vi "Load Configuration.vi"(8 "error in":errorcluster, 11 "Config path":path=path "C:/GitHub/OOP_OPC UA/Config/INI Config.ini") -> (0 "error out":errorcluster)   [LabVIEW 2021]
uses:
  Controls/Channels.ctl
  Controls/Instrument.ctl
  Controls/DUT.ctl
  <vilib>/Utility/config.llb/Read Key (String).vi
  <vilib>/Utility/config.llb/NI_LVConfig.lvlib
panel:
  out "data":T1[](array[typedef])
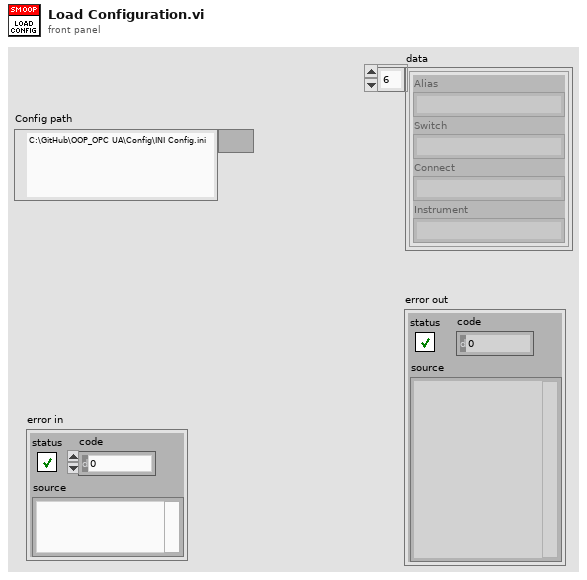
[diagram p1: front panel]
types:
  T1 = typedef "Channels.ctl" = cluster{"Alias":string, "Switch":string, "Connect":string, "Instrument":string}
  T2 = typedef "NI_LVConfig.lvlib/Config Data RefNum.ctl" = refnum<k1>
  T3 = typedef "Instrument.ctl" = cluster{"Alias":string, "VISA Resource":string, "Class":string}
  T4 = typedef "DUT.ctl" = cluster{"Alias":string, "Instrument":string, "Channel":string}
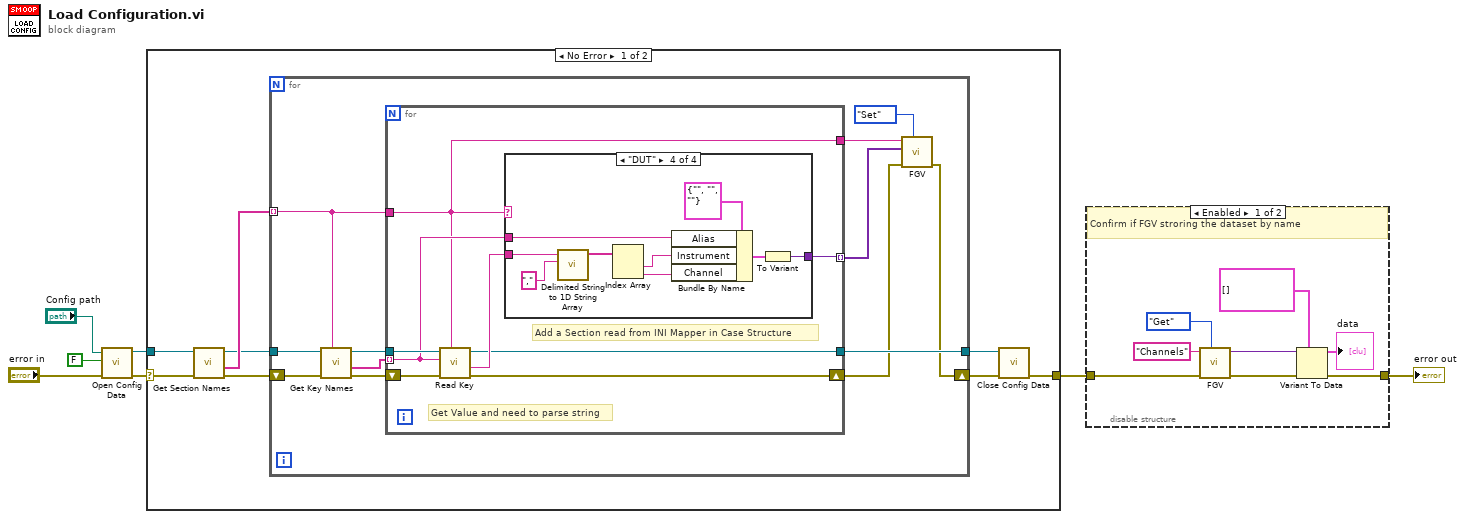
[diagram p0: block diagram]
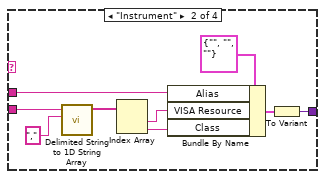
[diagram p3: hidden frame]
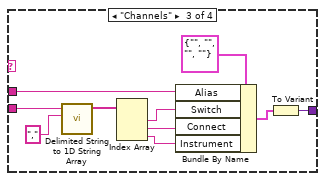
[diagram p4: hidden frame]
diagram:
  n1 = call <vilib>:"Open Config Data.vi"("error in (no error)"="error in", "create file if necessary (T)"=FALSE, "configuration file path"="Config path") -> ("error out"=w5:errorcluster, "refnum"=w6:T2)  [unwired: 6 in, 1 out]
  n2 = case shown="No Error" w5 {
    selector: w5 -> [w15 w64]
    tunnel: [w8 w64] -> w2
    tunnel: w6 -> [w14 _]
    frame No Error {
      n3 = call <vilib>:"Get Section Names.vi"("error in (no error)"=w15, "refnum"=w14) -> ("error out"=w12:errorcluster, "section names"=w13:string[], "refnum out"=w11:T2)  [unwired: 7 in]
      n4 = for {
        tunnel: w13 -> [w24] mode=indexing
        tunnel: w11 -> [w26]
        tunnel: [w25] -> w10
        shift-right: [w18] -> w9
        shift-left: w12 -> [w27]
        n5 = call <vilib>:"Get Key Names.vi"("section"=w24, "error in (no error)"=w27, "refnum"=w26) -> ("error out"=w23:errorcluster, "key names"=w22:string[], "refnum out"=w21:T2)  [unwired: 5 in, 1 out]
        n6 = for {
          tunnel: w22 -> [w32] mode=indexing
          tunnel: w24 -> [w28]
          tunnel: w21 -> [w34]
          tunnel: [w30] -> w25
          tunnel: [w29] -> w16 mode=indexing
          tunnel: [w28] -> w17
          shift-right: [w33] -> w19
          shift-left: w23 -> [w35]
          # "Add a Section read from INI Mapper in Case Structure"
          # "Get Value and need to parse string"
          n7 = call-poly <vilib>:"Read Key.vi"("section"=w28, "error in (no error)"=w35, "key"=w32, "refnum"=w34) -> ("error out"=w33:errorcluster, "value"=w31:string, "refnum out"=w30:T2)  [unwired: 4 in, 1 out]
          n8 = case shown="\"DUT\"" w28 {
            tunnel: w32 -> [_ w38 w48 w58]
            tunnel: w31 -> [_ w39 w49 w59]
            tunnel: [_ w36 w45 w55] -> w29
            frame Default {
            }
            frame "Instrument" {
              n9 = call <vilib>:"Delimited String to 1D String Array.vi"("delimiter"=",", "delimited string"=w39) -> ("string array"=w37:string[])  [unwired: 9 in]
              n10 = Index Array(array=w37) -> (element #1=w41:string, element #2=w40:string)  [unwired: 2 in]
              n11 = Bundle By Name(cluster=T3 {"Alias"="", "VISA Resource"="", "Class"=""} ("Instruments"), "Alias"=w38, "VISA Resource"=w41, "Class"=w40) -> (w43:T3)
              n12 = To Variant(anything=w43) -> (Variant=w36:variant)
            }
            frame "Channels" {
              n13 = call <vilib>:"Delimited String to 1D String Array.vi"("delimiter"=",", "delimited string"=w49) -> ("string array"=w52:string[])  [unwired: 9 in]
              n14 = Index Array(array=w52) -> (element #1=w51:string, element #2=w50:string, element #3=w46:string)  [unwired: 3 in]
              n15 = Bundle By Name(cluster=T1 {"Alias"="", "Switch"="", "Connect"="", "Instrument"=""} ("Channels"), "Alias"=w48, "Switch"=w51, "Connect"=w50, "Instrument"=w46) -> (w54:T1)
              n16 = To Variant(anything=w54) -> (Variant=w45:variant)
            }
            frame "DUT" {
              n17 = call <vilib>:"Delimited String to 1D String Array.vi"("delimiter"=",", "delimited string"=w59) -> ("string array"=w62:string[])  [unwired: 9 in]
              n18 = Index Array(array=w62) -> (element #1=w61:string, element #2=w60:string)  [unwired: 2 in]
              n19 = Bundle By Name(cluster=T4 {"Alias"="", "Instrument"="", "Channel"=""} ("DUT"), "Alias"=w58, "Instrument"=w61, "Channel"=w60) -> (w56:T4)
              n20 = To Variant(anything=w56) -> (Variant=w55:variant)
            }
          }
        }
        n21 = call "FGV.vi"("Method (Get)"=enum16{"Get", "Set"}."Set", "error in"=w19, "Data In"=w16, "Name"=w17) -> ("error out"=w18:errorcluster)  [unwired: 6 in, 1 out]
      }
      n22 = call <vilib>:"Close Config Data.vi"("error in (no error)"=w9, "refnum"=w10) -> ("error out"=w8:errorcluster)  [unwired: 8 in, 1 out]
    }
    frame Error {
    }
  }
  n23 = disable-structure "Diagram Disable Structure" shown="Enabled" {
    disable-tunnel: w2 -> [w72 w73]
    disable-tunnel: [w68 w73] -> w1
    frame Enabled {
      # "Confirm if FGV stroring the dataset by name"
      n24 = call "FGV.vi"("Method (Get)"=enum16{"Get", "Set"}."Get", "error in"=w72, "Name"="Channels") -> ("error out"=w70:errorcluster, "Data out"=w69:variant)  [unwired: 7 in]
      n25 = Variant To Data(error in=w70, type=T1[] [], Variant=w69) -> (data=→"data":T1[], error out=w68:errorcluster)
    }
    frame Disabled {
    }
  }
  "error out" <- w1
